vi "Test Write and Get Channel Reading.vi"(11 "Test Case In":refnum<class "Test BufferLossless.lvclass">) -> (0 "error out":errorcluster, 3 "Test Case Out":refnum<class "Test BufferLossless.lvclass">)   [LabVIEW 2024, in "Test BufferLossless.lvclass"]
uses:
  Test BufferLossless.lvclass
  C:/Program Files/National Instruments/LabVIEW 2024/vi.lib/Astemes/LUnit/Test Case.lvclass
  Devices/Buffers/BufferLossless/BufferLossless.lvclass
  <vilib>/Astemes/LUnit/Test Case.lvclass/Test Case.ctl
  4993e8ee-a06a-463a-9684-69129f64d5ce.vi
  <vilib>/Astemes/LUnit/Append Pass Result.vi
  <vilib>/Astemes/LUnit/Append Fail Result.vi
  <vilib>/Astemes/LUnit/Describe Comparison.vi
  4993e8ee-a06a-463a-9684-69129f64d5ce.vi/9c5d11cd-9439-4240-a1ee-d9baace9c924.vi
  <vilib>/Astemes/LUnit/Run In UI.vi
  <vilib>/Utility/error.llb/Clear Errors.vi
  <vilib>/Astemes/LUnit/Describe Variant.vi
  Test BufferLossless.lvclass/Test BufferLossless.ctl
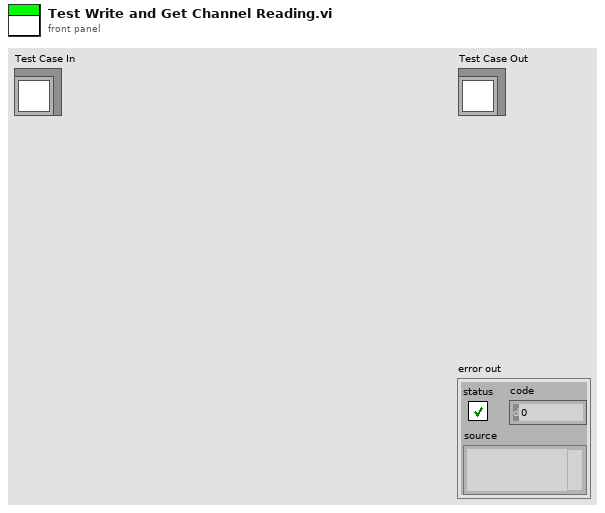
[diagram p1: front panel]
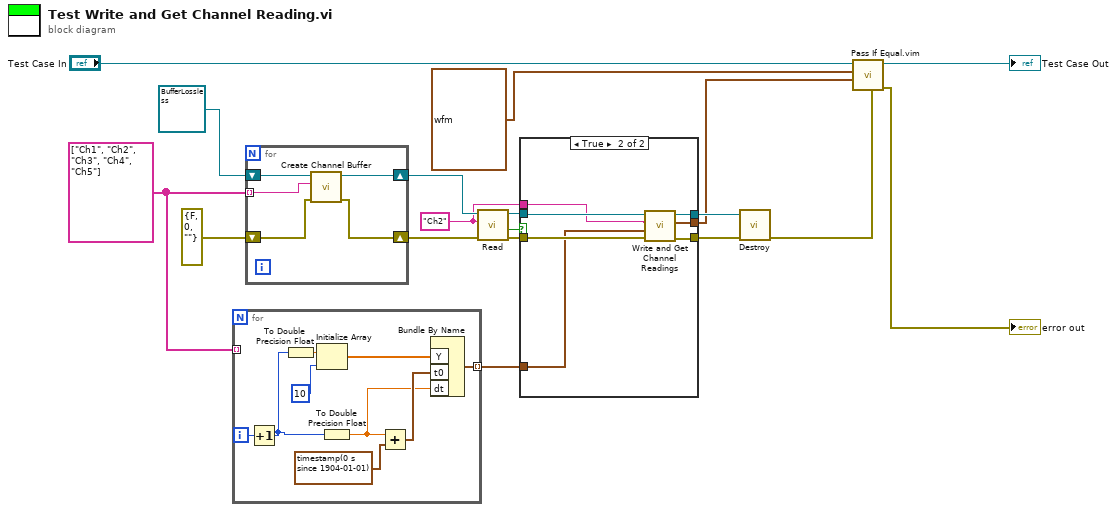
[diagram p0: block diagram]
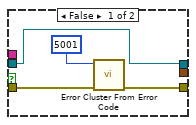
[diagram p2: hidden frame]
diagram:
  w8 = "Ch2"
  w7 = string[] ["Ch1", "Ch2", "Ch3", "Ch4", "Ch5"]
  n1 = for {
    tunnel: w7 -> [_] mode=indexing
    tunnel: [w20] -> w6 mode=indexing
    i -> [w24]
    n2 = Increment(x=w24) -> (x+1=w19:i32)
    n3 = To Double Precision Float(number=w19) -> (double precision float=w25:dbl)
    n4 = Initialize Array(w25, 10 ("dimension size")) -> (w26:dbl[])
    n5 = To Double Precision Float(number=w19) -> (double precision float=w21:dbl)
    n6 = Add(x=w21, y=timestamp(0 s since 1904-01-01) ("Time Stamp")) -> (x+y=w22:timestamp)
    n7 = Bundle By Name("Y"=w26, "t0"=w22, "dt"=w21) -> (w20:waveform(dbl))  [unwired: 1 in]
  }
  n8 = for {
    shift-right: [w28] -> w13
    shift-left: errorcluster {"status"=FALSE, "code"=0, "source"=""} ("error in (no error)") -> [w31]
    tunnel: w7 -> [w30] mode=indexing
    shift-right: [w29] -> w12
    shift-left: refnum<class "BufferLossless.lvclass"> refnum ("BufferLossless out") -> [w32]
    n9 = call "Create Channel Buffer.vi"("error in"=w31, "Channel"=w30, "BufferLossless in"=w32) -> ("error out"=w28:errorcluster, "BufferLossless out"=w29:refnum<class "BufferLossless.lvclass">)  [unwired: 7 in]
  }
  n10 = call "Read.vi"("error in"=w13, "Channel"=w8, "BufferLossless in"=w12) -> ("error out"=w11:errorcluster, "empty?"=w10:bool, "BufferLossless out"=w9:refnum<class "BufferLossless.lvclass">)  [unwired: 5 in, 1 out]
  n11 = case shown="True" w10 {
    tunnel: w11 -> [w36 w43]
    tunnel: w9 -> [w33 w42]
    tunnel: w8 -> [_ w41]
    tunnel: w6 -> [_ w40]
    tunnel: [w34 w39] -> w5
    tunnel: [_ w38] -> w2
    tunnel: [w33 w37] -> w4
    frame False {
      n12 = call <vilib>:"Error Cluster From Error Code.vi"("error in (no error)"=w36, "error code (0)"=5001) -> ("error out"=w34:errorcluster)  [unwired: 7 in]
    }
    frame True {
      n13 = call "Write and Get Channel Readings.vi"("error in"=w43, "Readings"=w40, "Channel"=w41, "BufferLossless in"=w42) -> ("error out"=w39:errorcluster, "Reading"=w38:waveform(dbl), "BufferLossless out"=w37:refnum<class "BufferLossless.lvclass">)  [unwired: 5 in]
    }
  }
  n14 = call "Destroy.vi"("error in"=w5, "BufferLossless in"=w4) -> ("error out"=w3:errorcluster)  [unwired: 8 in, 1 out]
  n15 = call "Pass If Equal.vim"("error in (no error)"=w3, "Actual"=w2, "Expected"=waveform(dbl) {"t0"=timestamp(2 s since 1904-01-01), "dt"=2.0, "Y"=[2.0, 2.0, 2.0, 2.0, 2.0, 2.0, 2.0, 2.0, 2.0, 2.0]} ("Reading"), "LUnit Test Case In"="Test Case In") -> ("error out"=→"error out":errorcluster, "LUnit Test Case Out"=→"Test Case Out":refnum<class "Test BufferLossless.lvclass">)  [unwired: 6 in]
